vi "msg_notifier.get.vi"(11 "client in":refnum<class "client.lvclass">) -> (2 "book notifier":refnum<notifier>, 3 "client out":refnum<class "client.lvclass">)   [LabVIEW 2020, in "client.lvclass"]
uses:
  client.lvclass
  shared/message--cluster.ctl
  shared/request--enum.ctl
  client.lvclass/client.ctl
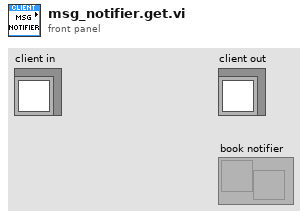
[diagram p1: front panel]
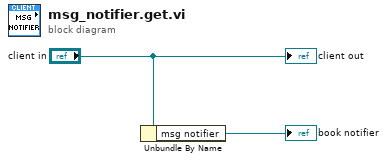
[diagram p0: block diagram]
diagram:
  n1 = Unbundle By Name("client in") -> ("msg notifier"=→"book notifier":refnum<notifier>)
  "client out" <- "client in"
